vi "SetLimit_axis.vi"(6 "max":dbl, 7 "min":dbl, 8 "error in (no error)":errorcluster, 9 "real pos zero":dbl, 10 "Axis":T1 items=["1"=1, "2"=2, "3"=3, "4"=4], 11 "DLOwis in":refnum<class "DLOwis.lvclass">) -> (0 "error out":errorcluster, 3 "DLOwis out":refnum<class "DLOwis.lvclass">)   [LabVIEW 2019, in "DLOwis.lvclass"]
uses:
  DLOwis.lvclass
  DelayLineLS4/LS4 axis.ctl
  DelayLine.lvclass
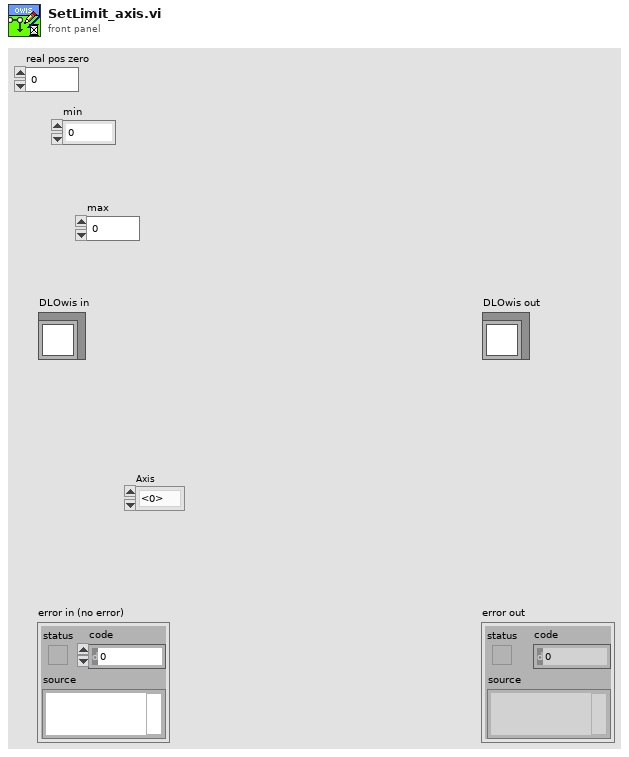
[diagram p1: front panel]
types:
  T1 = typedef "DelayLine.lvclass/LS4 axis.ctl" = u16
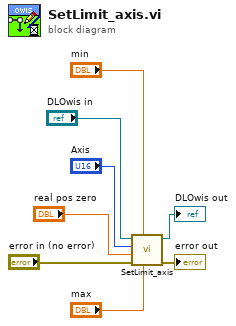
[diagram p0: block diagram]
diagram:
  n1 = call-parent "SetLimit_axis.vi"("max"="max", "min"="min", "error in (no error)"="error in (no error)", "real pos zero"="real pos zero", "Axis"="Axis", "DelayLine in"="DLOwis in") -> ("error out"=→"error out":errorcluster, "DelayLine out"=→"DLOwis out":refnum<class "DLOwis.lvclass">)  [unwired: 4 in]
